vi "Free_LaEW_Memory.vi"() -> (1 "Total Free (MB)":dbl format="%.2f", 2 "Largest Block Free (MB)":dbl format="%.2f")   [LabVIEW 2010]
uses:
  Globals/Preference_global.vi
panel:
  in  "AZ memStats In":T1
  out "AZ memStats":T1
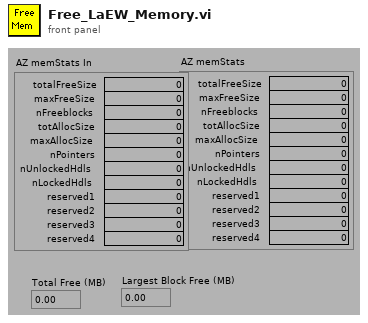
[diagram p1: front panel]
types:
  T1 = cluster{"totalFreeSize":i32, "maxFreeSize":i32, "nFreeblocks":i32, "totAllocSize":i32, "maxAllocSize":i32, "nPointers":i32, "nUnlockedHdls":i32, "nLockedHdls":i32, "reserved1":i32, "reserved2":i32, "reserved3":i32, "reserved4":i32}
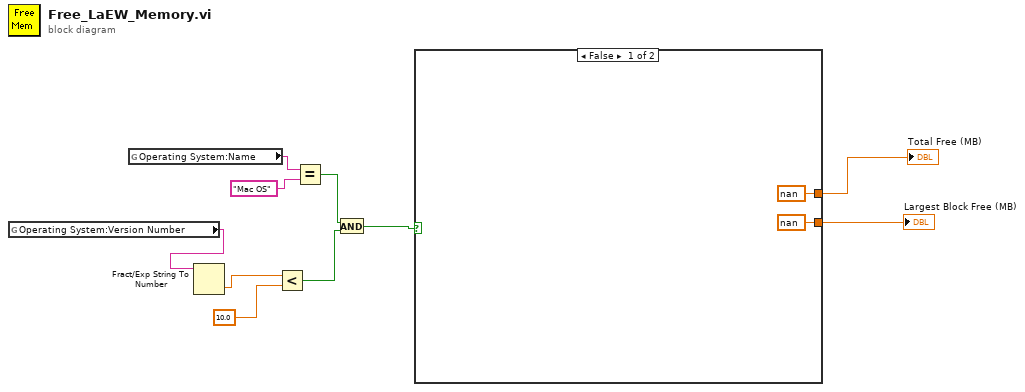
[diagram p0: block diagram]
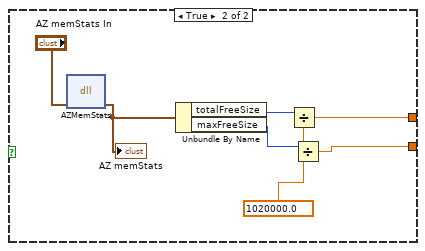
[diagram p2: hidden frame]
diagram:
  n1 = global read "Preference_global.vi" "Operating System:Version Number"() -> (w6:string)
  n2 = global read "Preference_global.vi" "Operating System:Name"() -> (w7:string)
  n3 = Fract/Exp String To Number(string=w6) -> (number=w5:dbl)  [unwired: 3 in, 1 out]
  n4 = Less?(x=w5, y=10.0) -> (x < y?=w3:bool)
  n5 = Equal?(x=w7, y="Mac OS" ("Operating System:Name")) -> (x = y?=w2:bool)
  n6 = And(x=w2, y=w3) -> (x .and. y?=w1:bool)
  n7 = case shown="False" w1 {
    tunnel: [nan w16] -> w10
    tunnel: [nan w13] -> w9
    frame False {
    }
    frame True {
      w14 = 1020000.0 ("y")
      n8 = dll-call lib="LabVIEW" fn="AZMemStats"("AZ memStats In"="AZ memStats In") -> ("AZ memStats In"=w19:T1)  [unwired: 4 in, 2 out]
      "AZ memStats" <- w19
      n9 = Unbundle By Name(w19) -> ("totalFreeSize"=w18:i32, "maxFreeSize"=w15:i32)
      n10 = Divide(x=w18, y=w14) -> (x/y=w16:dbl)
      n11 = Divide(x=w15, y=w14) -> (x/y=w13:dbl)
    }
  }
  "Total Free (MB)" <- w10
  "Largest Block Free (MB)" <- w9
